vi "Get SA Pin.vi"(8 "error in (no error)":errorcluster, 11 "SPECAN_PVT in":refnum<class "SPECAN_PVT.lvclass">) -> (0 "error out":errorcluster, 2 "SA PIN":string, 3 "SPECAN_PVT out":refnum<class "SPECAN_PVT.lvclass">)   [LabVIEW 2018, in "SPECAN_PVT.lvlib" / "SPECAN_PVT.lvclass"]
uses:
  SPECAN_PVT.lvclass
  C:/Sequence Automation/Plugins/Measurement Interface.lvlibp/Measurement Interface.lvclass
  Plugins/Measurement Interface.lvlibp/Private Methods/Measurement Parameters/Read Measurement Parameters.vi
  Plugins/String Database.lvlibp/String Database.lvclass
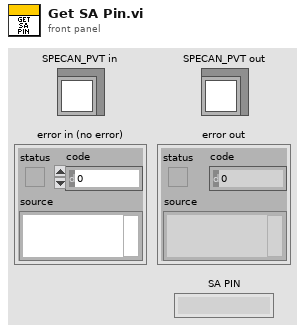
[diagram p1: front panel]
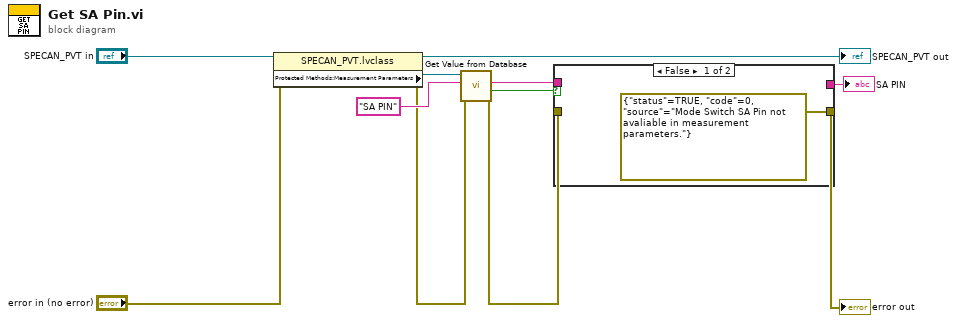
[diagram p0: block diagram]
diagram:
  n1 = property class="SPECAN_PVT.lvclass"(reference="SPECAN_PVT in", error in="error in (no error)") -> (reference out=→"SPECAN_PVT out":refnum<class "SPECAN_PVT.lvclass">, error out=w9:errorcluster, "Protected Methods:Measurement Parameters"=w11:refnum<class "String Database.lvclass">)
  n2 = call "Get Value from Database.vi"("error in (no error)"=w9, "Entry Name"="SA PIN", "Message in"=w11) -> ("error out"=w7:errorcluster, "Entry Found"=w8:bool, "Entry Value"=w6:string)  [unwired: 5 in, 1 out]
  n3 = case shown="False" w8 {
    tunnel: w7 -> [_ w13]
    tunnel: [errorcluster {"status"=TRUE, "code"=0, "source"="Mode Switch SA Pin not avaliable in measurement parameters."} ("error out") w13] -> w3
    tunnel: w6 -> [_ w14]
    tunnel: [_ w14] -> w1
    frame False {
    }
    frame True {
    }
  }
  "error out" <- w3
  "SA PIN" <- w1
